vi "DisableSteppers.vi"(8 "error in (no error)":errorcluster caption="Fehler (Eingang, kein Fehler)", 11 "Moveo Eingang":refnum<class "Moveo.lvclass">) -> (0 "error out":errorcluster caption="Fehler (Ausgang)", 3 "Moveo Ausgang":refnum<class "Moveo.lvclass">)   [LabVIEW 2019, in "Moveo.lvclass"]
uses:
  Moveo.lvclass
  Moveo.lvclass/Moveo.ctl
  MoveoSerialClass/MoveoSerial.lvclass
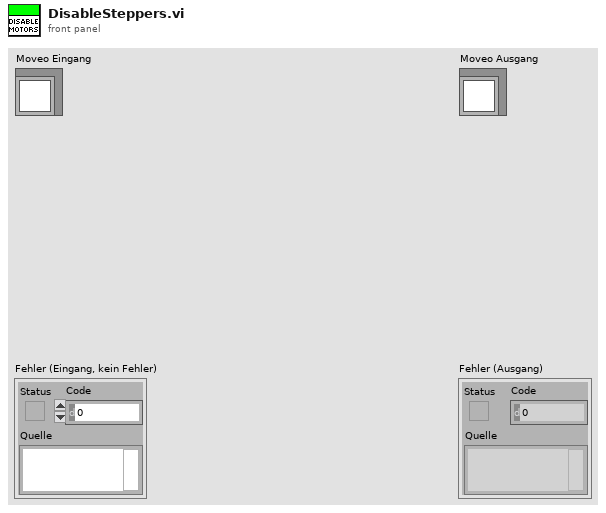
[diagram p1: front panel]
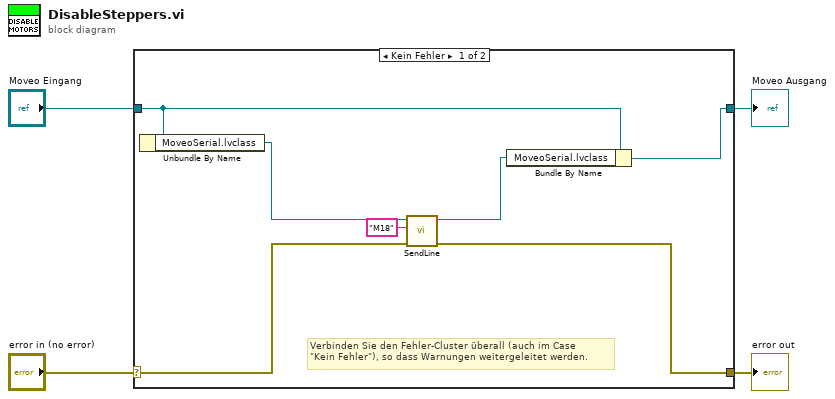
[diagram p0: block diagram]
diagram:
  n1 = case shown="Kein Fehler" "error in (no error)" {
    selector: "error in (no error)" -> [w10 w13]
    tunnel: [w9 w13] -> w3
    tunnel: [w7 w12] -> w1
    tunnel: "Moveo Eingang" -> [w8 w12]
    frame No Error {
      # "Verbinden Sie den Fehler-Cluster überall (auch im Case\n\"Kein Fehler\"), so dass Warnungen weitergeleitet werden."
      n2 = Unbundle By Name(w8) -> ("MoveoSerial.lvclass"=w11:refnum<class "MoveoSerial.lvclass">)
      n3 = call-dynamic "SendLine.vi"("error in (no error)"=w10, "SendString"="M18", "MoveoSerial Eingang"=w11) -> ("error out"=w9:errorcluster, "MoveoSerial Ausgang"=w6:refnum<class "MoveoSerial.lvclass">)  [unwired: 7 in]
      n4 = Bundle By Name(cluster=w8, "MoveoSerial.lvclass"=w6) -> (w7:refnum<class "Moveo.lvclass">)
    }
    frame Error {
    }
  }
  "error out" <- w3
  "Moveo Ausgang" <- w1
